vi "Not In Unified Msg Set.vi"(11 "Base Actor in":refnum<class "Base Actor.lvclass">) -> (0 "Error out":errorcluster, 3 "Base Actor out":refnum<class "Base Actor.lvclass">)   [LabVIEW 2025, in "jettl.lvlib" / "Actor.lvlib" / "Base Actor.lvclass"]
uses:
  Base Actor.lvclass
  Base Actor.lvclass/Base Actor.ctl
  Error/Error.lvlib
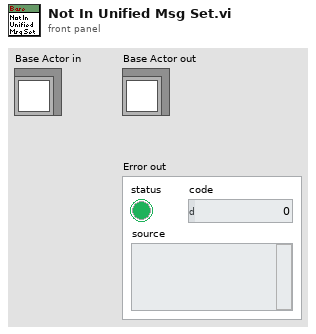
[diagram p1: front panel]
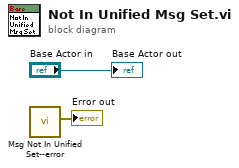
[diagram p0: block diagram]
diagram:
  n1 = call "Msg Not In Unified Set--error.vi"() -> ("Error"=→"Error out":errorcluster)  [unwired: 11 in]
  "Base Actor out" <- "Base Actor in"
